vi "TDMS0_ECD.vi"(2 "Startmethode":i32, 3 "Dateiname":string, 4 "Dateiordner":path) -> (0 "tdms1":refnum<k34>, 1 "tdms0":refnum<k34>)   [LabVIEW 2017]
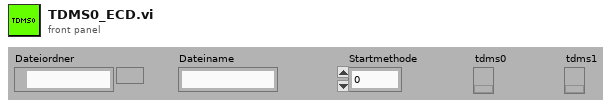
[diagram p1: front panel]
types:
  T1 = enum16{"open", "open or create", "create or replace", "create", "open (read-only)"}
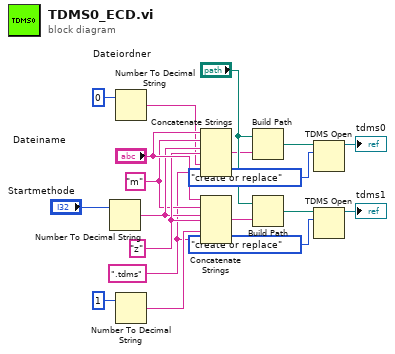
[diagram p0: block diagram]
diagram:
  w12 = "z"
  w10 = "m"
  w9 = ".tdms" ("String")
  n1 = Number To Decimal String(number="Startmethode") -> (decimal integer string=w11:string)  [unwired: 1 in]
  n2 = Number To Decimal String(number=0 ("Wert")) -> (decimal integer string=w8:string)  [unwired: 1 in]
  n3 = Number To Decimal String(number=1 ("Wert")) -> (decimal integer string=w13:string)  [unwired: 1 in]
  n4 = Concatenate Strings("Dateiname", w10, w11, w12, w8, w9) -> (w4:string)
  n5 = Concatenate Strings("Dateiname", w10, w11, w12, w13, w9) -> (w5:string)
  n6 = Build Path(base path="Dateiordner", name or relative path=w4) -> (appended path=w3:path)
  n7 = Build Path(base path="Dateiordner", name or relative path=w5) -> (appended path=w14:path)
  n8 = TDMS Open(10:T1."create or replace" ("Operation (0:Öffnen)"), 11:w3) -> (3:→"tdms0":refnum<k34>)  [unwired: 5 in, 1 out]
  n9 = TDMS Open(10:T1."create or replace" ("Operation (0:Öffnen)"), 11:w14) -> (3:→"tdms1":refnum<k34>)  [unwired: 5 in, 1 out]
